vi "Build Trianary array.vi"(7 "Size":i32, 11 "itteration":i32) -> (3 "output array":i32[](array[numeric]))   [LabVIEW 2024]
uses:
  99fa8f46-1761-4833-8f3d-fa6f00eab163.vi
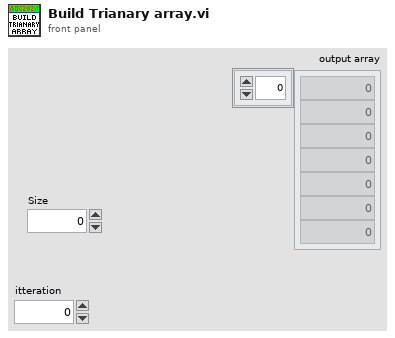
[diagram p1: front panel]
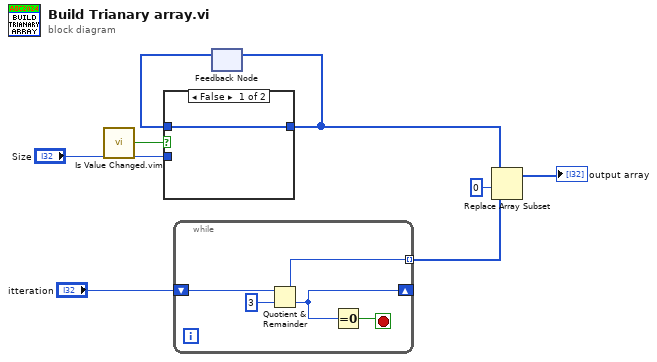
[diagram p0: block diagram]
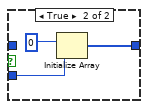
[diagram p2: hidden frame]
diagram:
  n1 = call "Is Value Changed.vim"("value"="Size") -> ("changed or first call?"=w7:bool)
  n2 = while {
    shift-right: [w10] -> _
    shift-left: "itteration" -> [w13]
    tunnel: [w11] -> w3 mode=indexing
    stop <- w9 stop-if-true
    n3 = Quotient & Remainder(x=w13, y=3) -> (x-y*floor(x/y)=w11:i32, floor(x/y)=w10:i32)
    n4 = Equal To 0?(x=w10) -> (x = 0?=w9:bool)
  }
  n5 = feedback #1() -> (w4:i32[])  [unwired: 1 in]
  n6 = case shown="False" w7 {
    tunnel: "Size" -> [_ w16]
    tunnel: [w14 w15] -> w5
    tunnel: w4 -> [w14 _]
    frame False {
    }
    frame True {
      n7 = Initialize Array(0 ("x-y*floor(x/y)"), w16) -> (w15:i32[])
    }
  }
  n8 = feedback-in #1(w5) -> ()
  n9 = Replace Array Subset(array=w5, new element=w3, index=0) -> (→"output array":i32[])
